vi "服务器端.vi"() -> ()   [LabVIEW 2020]
uses:
  65fd9499-b6d8-44bb-ab61-33a386fe496d.vi
  31329c15-849f-4aa1-ac13-bc2ee6c68659.vi
panel:
  out "连接数量":i32
  out "错误输出":errorcluster
  in  "发送按钮":bool
  in  "停止":bool
  out "接收信息":string
  in  "发送信息":string
  out "创建成功指示":bool
  in  "端口":u16
  in  "IP":string
  in  "创建按钮":bool
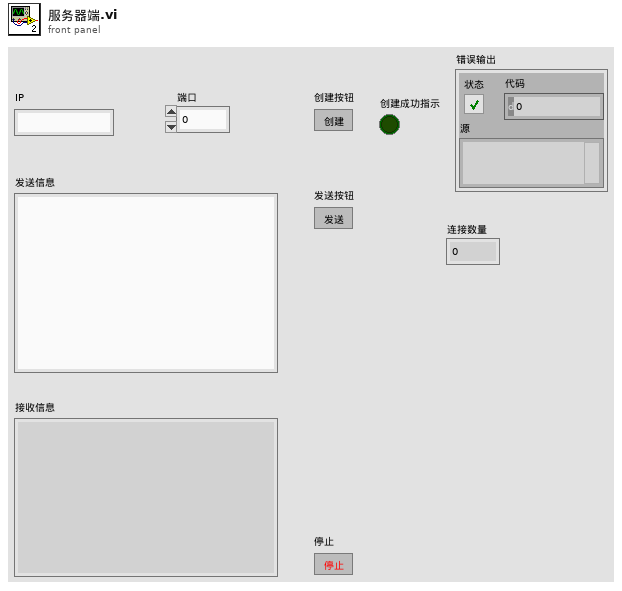
[diagram p1: front panel]
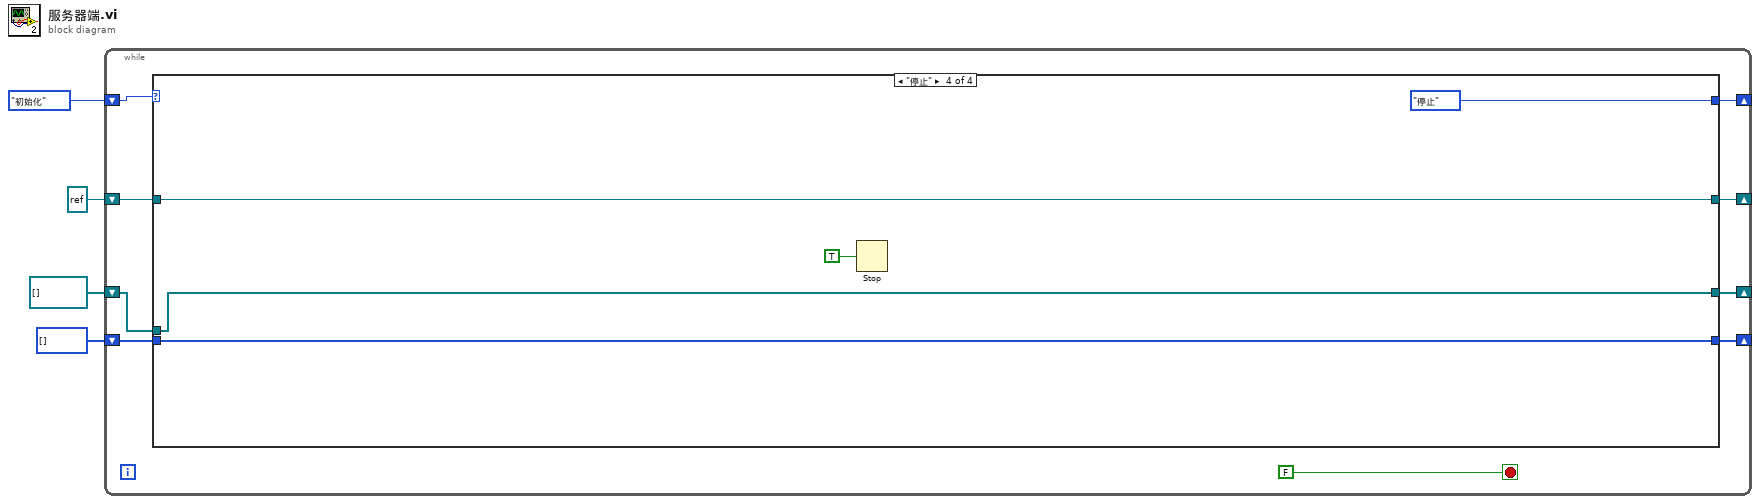
[diagram p0: block diagram]
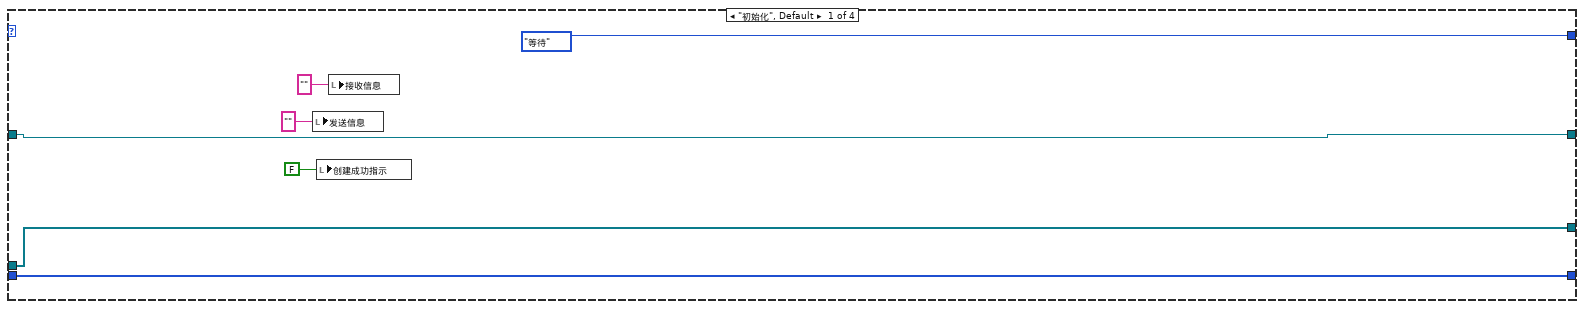
[diagram p2: hidden frame]
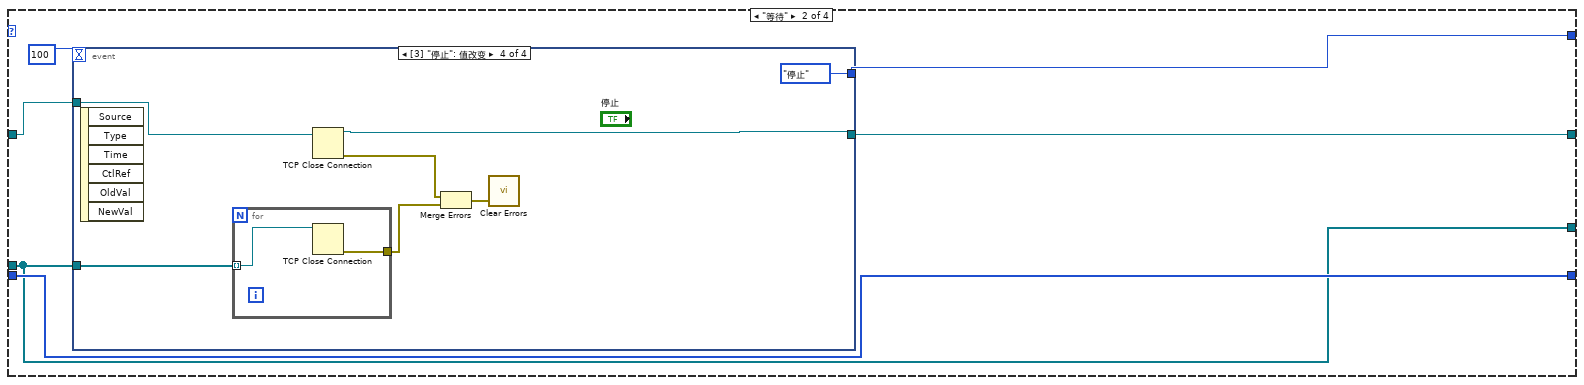
[diagram p3: hidden frame]
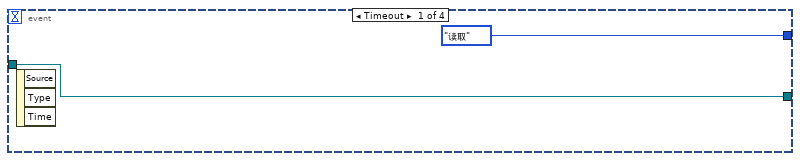
[diagram p4: hidden frame]
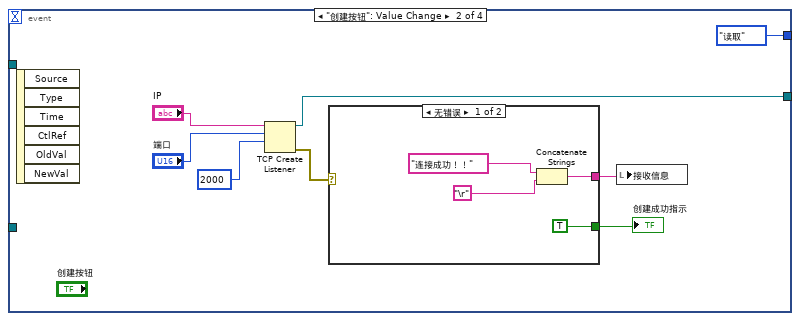
[diagram p5: hidden frame]
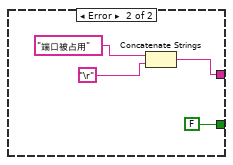
[diagram p6: hidden frame]
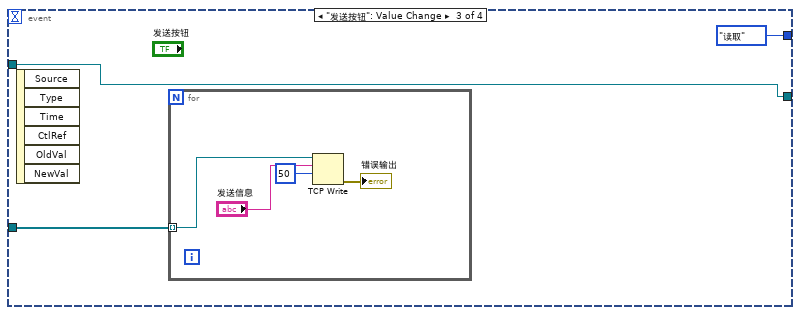
[diagram p7: hidden frame]
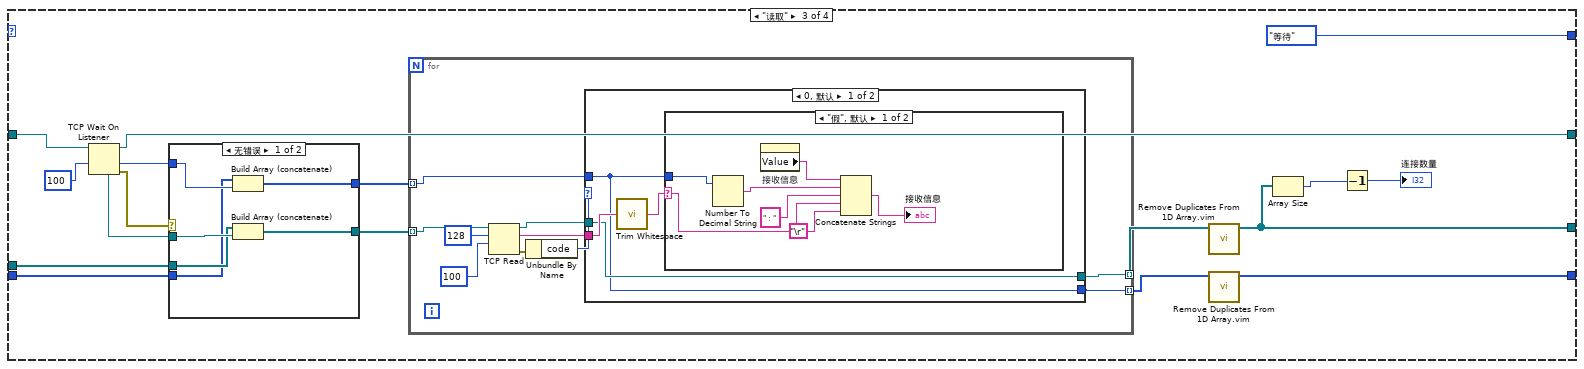
[diagram p8: hidden frame]
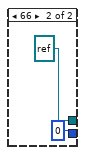
[diagram p10: hidden frame]
diagram:
  n1 = while {
    shift-right: [w11] -> _
    shift-left: enum16{"初始化", "等待", "读取", "停止"}."初始化" -> [w12]
    shift-right: [w10] -> _
    shift-left: refnum<k5> refnum ("listener ID") -> [w9]
    shift-right: [w8] -> _
    shift-left: refnum<k5>[] [] ("array with duplicates removed") -> [w6]
    shift-right: [w7] -> _
    shift-left: u16[] [] ("array with duplicates removed") -> [w5]
    stop <- FALSE stop-if-true
    n2 = case shown="\"停止\"" w12 {
      tunnel: [enum16{"初始化", "等待", "读取", "停止"}."等待" w25 enum16{"初始化", "等待", "读取", "停止"}."等待" enum16{"初始化", "等待", "读取", "停止"}."停止"] -> w11
      tunnel: [w16 w24 w75 w111] -> w10
      tunnel: w9 -> [w16 w23 w77 w111]
      tunnel: [w15 w21 w63 w113] -> w8
      tunnel: [w14 w22 w67 w112] -> w7
      tunnel: w6 -> [w15 w21 w66 w113]
      tunnel: w5 -> [w14 w22 w65 w112]
      frame "初始化", Default {
        n3 = local write "发送信息"("" ("发送信息")) -> ()
        n4 = local write "创建成功指示"(FALSE ("创建成功指示")) -> ()
        n5 = local write "接收信息"("" ("接收信息")) -> ()
      }
      frame "等待" {
        n6 = event shown="[3] \"停止\": 值改变" {
          selector: _ -> [_ _ _ _]
          dyn-events: _ -> [_ _ _ _]
          timeout: 100 -> [_ _ _ _]
          tunnel: [enum16{"初始化", "等待", "读取", "停止"}."读取" enum16{"初始化", "等待", "读取", "停止"}."读取" enum16{"初始化", "等待", "读取", "停止"}."读取" enum16{"初始化", "等待", "读取", "停止"}."停止"] -> w25
          tunnel: [w27 w29 w47 w54] -> w24
          tunnel: w23 -> [w27 _ w47 w58]
          tunnel: w21 -> [_ _ w45 w52]
          event Timeout {
            n7 = event-data() -> ()  [unwired: 1 in, 3 out]
          }
          event "创建按钮": Value Change {
            n8 = event-data() -> ()  [unwired: 1 in, 6 out]
            n9 = TCP Create Listener(9:2000 ("超时毫秒(25000)"), 10:"端口", 11:"IP") -> (0:w33:errorcluster, 3:w29:refnum<k5>)  [unwired: 2 in, 1 out]
            n10 = case shown="无错误" w33 {
              tunnel: [TRUE FALSE] -> w32
              tunnel: [w37 w41] -> w31
              frame No Error {
                n11 = Concatenate Strings("连接成功！！", "\r") -> (w37:string)
              }
              frame Error {
                n12 = Concatenate Strings("端口被占用", "\r") -> (w41:string)
              }
            }
            "创建成功指示" <- w32
            n13 = local write "接收信息"(w31) -> ()
          }
          event "发送按钮": Value Change {
            n14 = event-data() -> ()  [unwired: 1 in, 6 out]
            n15 = for {
              tunnel: w45 -> [w49] mode=indexing
              n16 = TCP Write(connection ID=w49, data in="发送信息", 9:50 ("超时毫秒(25000)")) -> (error out=→"错误输出":errorcluster)  [unwired: 1 in, 2 out]
            }
          }
          event "停止": Value Change {
            n17 = event-data() -> ()  [unwired: 1 in, 6 out]
            n18 = for {
              tunnel: [w60] -> w57
              tunnel: w52 -> [w59] mode=indexing
              n19 = TCP Close Connection(connection ID=w59) -> (error out=w60:errorcluster)  [unwired: 2 in, 1 out]
            }
            n20 = TCP Close Connection(connection ID=w58) -> (connection ID out=w54:refnum<k5>, error out=w56:errorcluster)  [unwired: 2 in]
            n21 = Merge Errors(w56, w57) -> (w55:errorcluster)
            n22 = call <vilib>:"Clear Errors.vi"("error in (no error)"=w55) -> ()  [unwired: 5 in, 2 out]
          }
        }
      }
      frame "读取" {
        n23 = TCP Wait On Listener(9:100 ("超时毫秒（一直等待:-1）"), 11:w77) -> (0:w74:errorcluster, 1:w73:u16, 3:w75:refnum<k5>, 4:w72:refnum<k5>)  [unwired: 2 in, 1 out]
        n24 = case shown="无错误" w74 {
          tunnel: w73 -> [w106 _]
          tunnel: w72 -> [w105 _]
          tunnel: [w104 w108] -> w71
          tunnel: [w103 w107] -> w70
          tunnel: w66 -> [w102 w108]
          tunnel: w65 -> [w101 w107]
          frame No Error {
            n25 = Build Array (concatenate)(w101, w106) -> (w103:u16[])
            n26 = Build Array (concatenate)(w102, w105) -> (w104:refnum<k5>[])
          }
          frame Error {
          }
        }
        n27 = for {
          tunnel: w71 -> [w87] mode=indexing
          tunnel: w70 -> [w80] mode=indexing
          tunnel: [w79] -> w69 mode=indexing
          tunnel: [w78] -> w68 mode=indexing
          n28 = TCP Read(connection ID=w87, bytes to read=128 ("读取的字节"), 9:100 ("超时毫秒(25000)")) -> (connection ID out=w81:refnum<k5>, data out=w82:string, error out=w84:errorcluster)  [unwired: 2 in]
          n29 = Unbundle By Name(w84) -> ("code"=w83:i32)
          n30 = case shown="0, 默认" w83 {
            tunnel: w82 -> [w91 _]
            tunnel: w81 -> [w89 _]
            tunnel: w80 -> [w88 _]
            tunnel: [w89 refnum<k5> refnum ("listener ID")] -> w79
            tunnel: [w88 u16 0 ("remote port")] -> w78
            frame 0, Default {
              n31 = call <vilib>:"Trim Whitespace.vi"("string"=w91) -> ("trimmed string"=w90:string)  [unwired: 1 in]
              n32 = case shown="\"假\", 默认" w90 {
                selector: w90 -> [w94 _]
                tunnel: w88 -> [w98 _]
                frame "假", Default {
                  n33 = Number To Decimal String(number=w98) -> (decimal integer string=w96:string)  [unwired: 1 in]
                  n34 = property on="接收信息" class="Str"() -> ("Value"=w97:string)  [unwired: 2 in, 2 out]
                  n35 = Concatenate Strings(w97, w96, "：", w94, "\r") -> (→"接收信息":string)
                }
                frame "" {
                }
              }
            }
            frame 66 {
            }
          }
        }
        n36 = call "Remove Duplicates From 1D Array.vim"("array"=w69) -> ("array with duplicates removed"=w63:refnum<k5>[])  [unwired: 10 in]
        n37 = call "Remove Duplicates From 1D Array.vim"("array"=w68) -> ("array with duplicates removed"=w67:u16[])  [unwired: 10 in]
        n38 = Array Size(array=w63) -> (size(s)=w62:i32)
        n39 = Decrement(x=w62) -> (x-1=→"连接数量":i32)
      }
      frame "停止" {
        n40 = Stop(stop? (T)=TRUE ("停止？(T)")) -> ()
      }
    }
  }
